vi "Pop Up.vi"(11 "Dev Actor in":refnum<class "Dev Actor.lvclass">) -> (3 "Dev Actor out":refnum<class "Dev Actor.lvclass">)   [LabVIEW 2021, in "Dev Actor.lvlib" / "Dev Actor.lvclass"]
uses:
  Dev Actor.lvclass
  C:/git/jettl/src/Queue Actor/Queue Actor.lvclass
  Dev Actor.lvclass/Dev Actor.ctl
  <vilib>/numeric/Random Number (Range) U64.vi
  <vilib>/numeric/sub_Random U32.vi
  Actor/Msgs/Create/Create Msg/Create Msg.lvclass
  C:/git/jettl/src/Actor/Msg/Msg.lvclass
  String Indicator Ref/String Indicator Ref/String Indicator Ref.lvclass
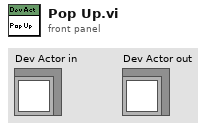
[diagram p1: front panel]
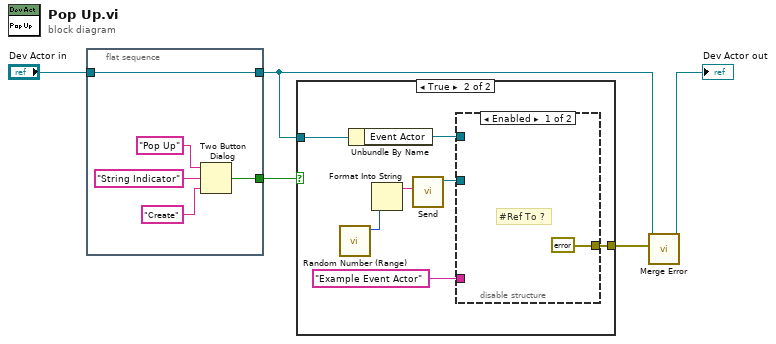
[diagram p0: block diagram]
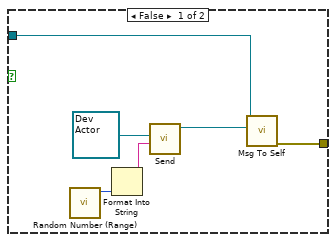
[diagram p2: hidden frame]
diagram:
  n1 = flat-sequence {
    tunnel: [w10] -> w1
    tunnel: "Dev Actor in" -> [w10]
    tunnel: [w7] -> w4
    frame #0 {
      n2 = Two Button Dialog(message="Pop Up", 1:"Create" ("F button name (\"Cancel\")"), 2:"String Indicator" ("T button name (\"OK\")")) -> (T button?=w7:bool)
    }
  }
  n3 = case shown="True" w4 {
    tunnel: w1 -> [w12 w23]
    tunnel: [w11 w18] -> w2
    frame False {
      n4 = call-poly <vilib>:"Random Number (Range).vi"() -> ("number"=w15:u64)  [unwired: 11 in]
      n5 = Format Into String(w15) -> (resulting string=w14:string)  [unwired: 3 in, 1 out]
      n6 = call "Send.vi"("Alias"=w14, "Queue Actor"=refnum<class "Dev Actor.lvclass"> refnum ("Dev Actor.lvlib:Dev Actor.lvclass")) -> ("Create Msg out"=w13:refnum<class "Create Msg.lvclass">)  [unwired: 9 in]
      n7 = call-dynamic "Msg To Self.vi"("Msg"=w13, "Dev Actor in"=w12) -> ("error out"=w11:errorcluster)  [unwired: 9 in]
    }
    frame True {
      n8 = call-poly <vilib>:"Random Number (Range).vi"() -> ("number"=w22:u64)  [unwired: 11 in]
      n9 = Unbundle By Name(w23) -> ("Event Actor"=w20:refnum<class "Event Actor.lvclass">)
      n10 = Format Into String(w22) -> (resulting string=w21:string)  [unwired: 3 in, 1 out]
      n11 = call "Send.vi"("String Indicator"=w21) -> ("String Indicator Ref out"=w19:refnum<class "String Indicator Ref.lvclass">)  [unwired: 10 in]
      n12 = disable-structure shown="Enabled" {
        disable-tunnel: w20 -> [_ _]
        disable-tunnel: w19 -> [_ _]
        disable-tunnel: [errorcluster {"status"=FALSE, "code"=0, "source"=""} ("error out") _] -> w18
        disable-tunnel: "Example Event Actor" -> [_ _]
        frame Enabled {
          # "#Ref To ?"
        }
        frame Disabled {
        }
      }
    }
  }
  n13 = call-dynamic "Merge Error.vi"("Error"=w2, "Dev Actor in"=w1) -> ("Dev Actor out"=→"Dev Actor out":refnum<class "Dev Actor.lvclass">)  [unwired: 9 in]
